vi "StateLED.vi"(0 "Master State In":T1(ring)) -> ()   [LabVIEW 2023]
doc: "This VI manages the apperance of the LEDs. The LED coloration and blink pattern report the robot mode and status. See project documentation for details."
uses:
  <vilib>/Rock Robotics/WPI/DriverStation/WPI_DriverStationRobotMode2.ctl
  GlobalMiscellaneous.vi
  GlobalDriverStationData.vi
  GlobalNoteHandling.vi
  GlobalElevator.vi
  GlobalShooter.vi
  GlobalDrivebase.vi
  GlobalAutonomous.vi
  GlobalPoseAndTargeting.vi
  <vilib>/vision/NI_Vision_Development_Module.lvlib
panel:
  in  "Shooter Ready Indication color":u32(colorbox)
  in  "Climb Background":u32(colorbox)=16717311
  in  "Speaker Background":u32(colorbox)=16717311
  in  "Amp Background":u32(colorbox)=16717311
  in  "Stow Background":u32(colorbox)=16717311
  in  "Human Control":u32(colorbox)=65280
  in  "Master Caution":u32(colorbox)=16736256
  in  "User Value Choice":u8(slide)=255 step=1 scale=0.0..255.0
  in  "User Saturation Choice":u8(slide)=255 step=1 scale=0.0..255.0
  in  "Pressure Insert":u32(colorbox)=91
  in  "Battery Insert":u32(colorbox)=65282
  in  "Pressure Background":u32(colorbox)=16711680
  in  "Battery Background":u32(colorbox)=16711680
  in  "Pressure LED Length":i32=6
  in  "Battery LED Length":i32=6
  in  "Battery Index":i32=4
  in  "Pressure Index":i32=4
  in  "Swerve 2 LED Index":i32
  in  "Swerve 3 LED Index":i32
  in  "Swerve 0 LED Index":i32=18
  in  "Swerve LED Length":i32=2
  in  "Swerve 1 LED Index":i32=18
  in  "Locate LED":bool
  in  "LED Index":i32
  out "User Blue":u8
  out "User Green":u8=255
  out "User Red":u8
  in  "Choose Hue":bool
  in  "User Hue Choice":u8(slide)=255 step=1 scale=0.0..255.0
  in  "Nominal":u32(colorbox)=65280
  in  "Master Alarm":u32(colorbox)=16711680
  in  "Robot Control":u32(colorbox)=16727040
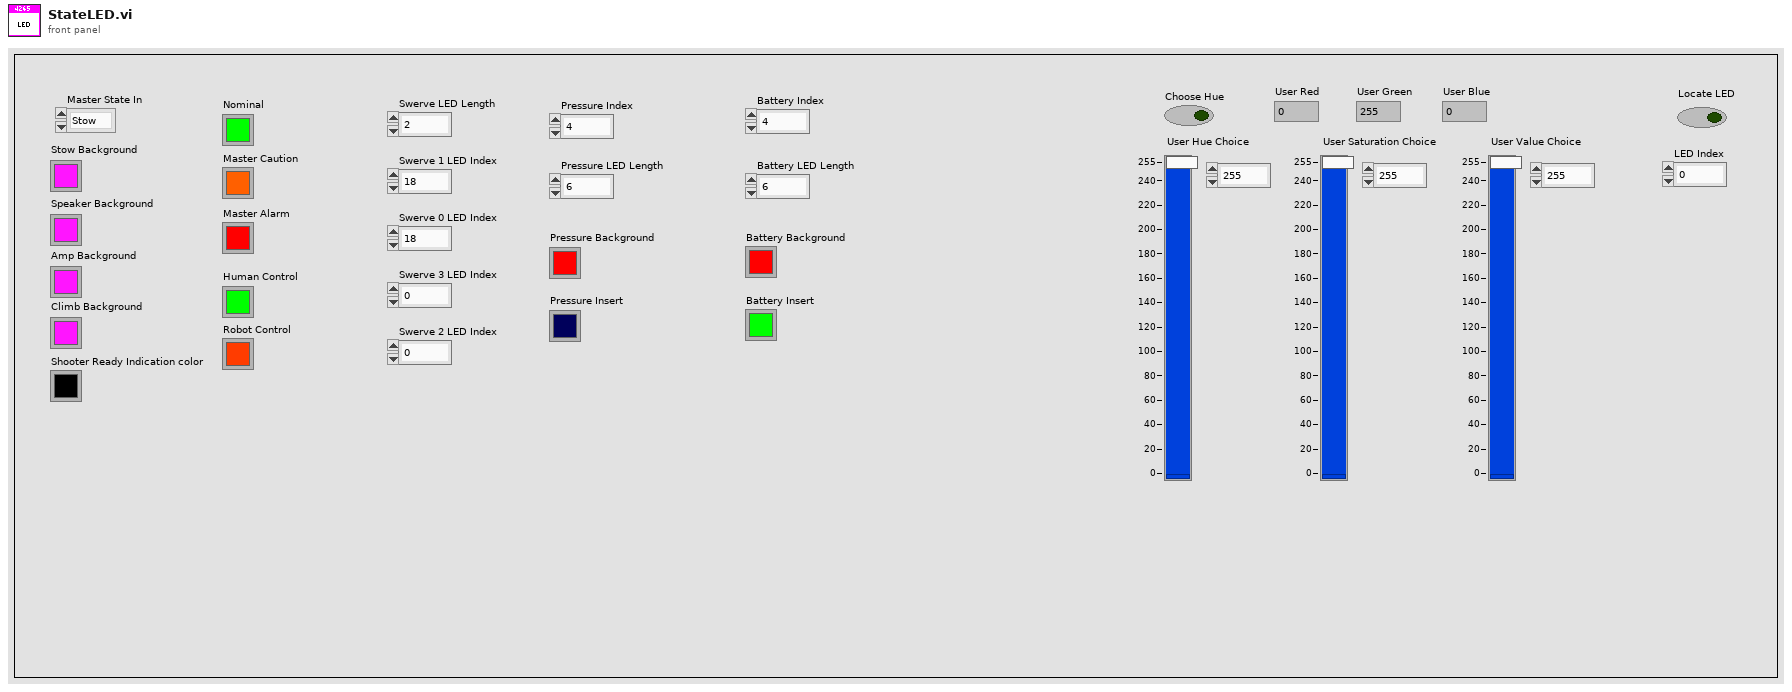
[diagram p1: front panel]
types:
  T1 = enum16{"Stow", "Speaker", "Amp", "Climbing", "Trap"}
  T2 = enum16{"Normal", "Party Mode", "Choose Hue", "Debug", "Locate LED", "Distance Rainbow"}
  T3 = typedef "WPI_DriverStationRobotMode2.ctl" = enum16{"Autonomous Disabled", "Autonomous Enabled", "Teleop Disabled", "Teleop Enabled", "Disconnected", "Finish", "Test Disabled", "Test Enabled", "Emergency Stopped"}
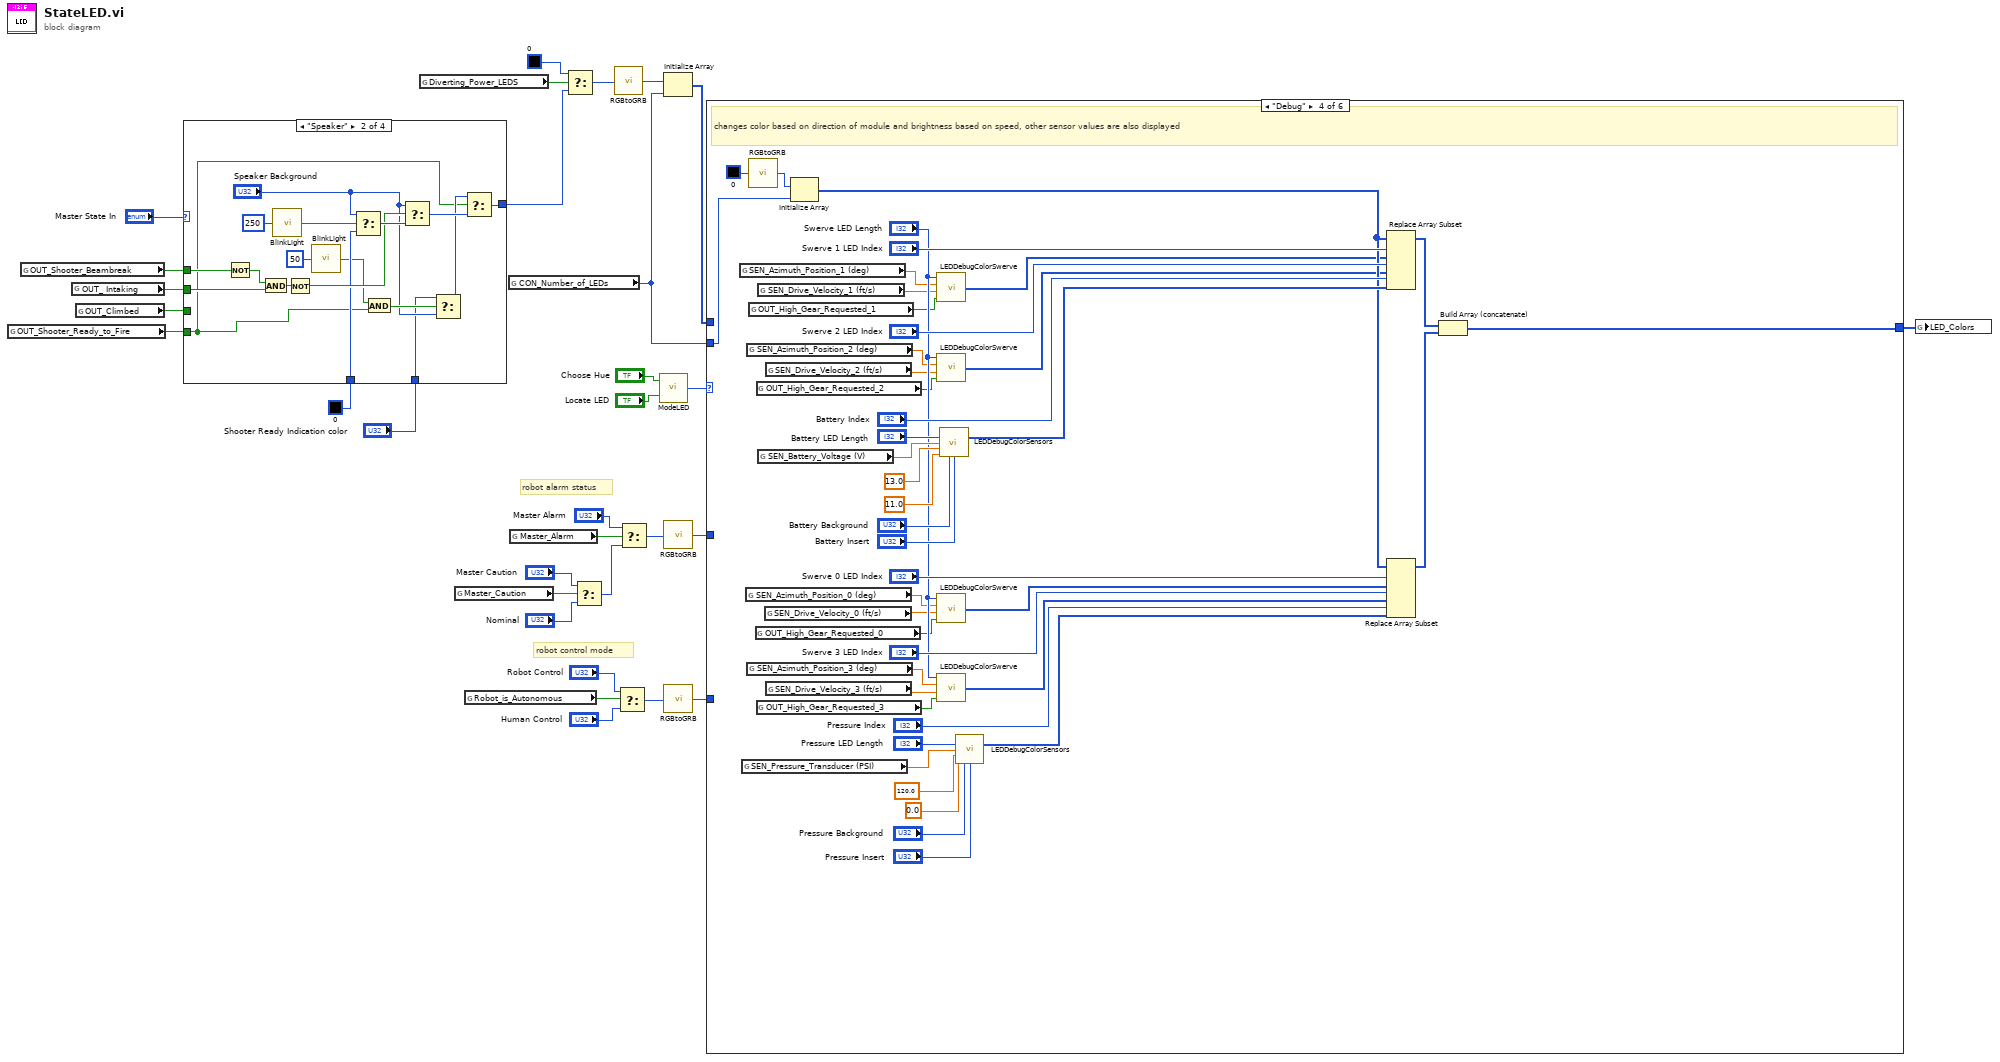
[diagram p0: block diagram]
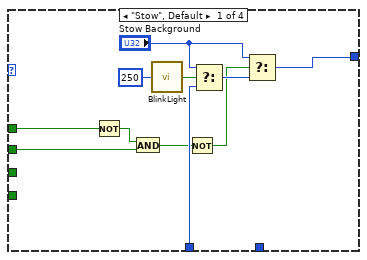
[diagram p2: hidden frame]
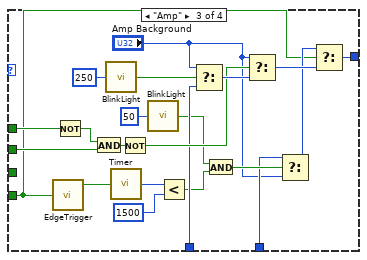
[diagram p3: hidden frame]
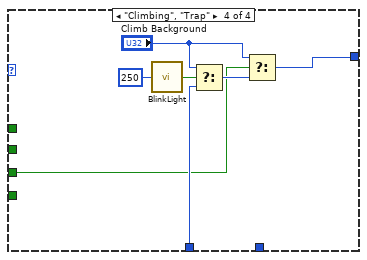
[diagram p4: hidden frame]
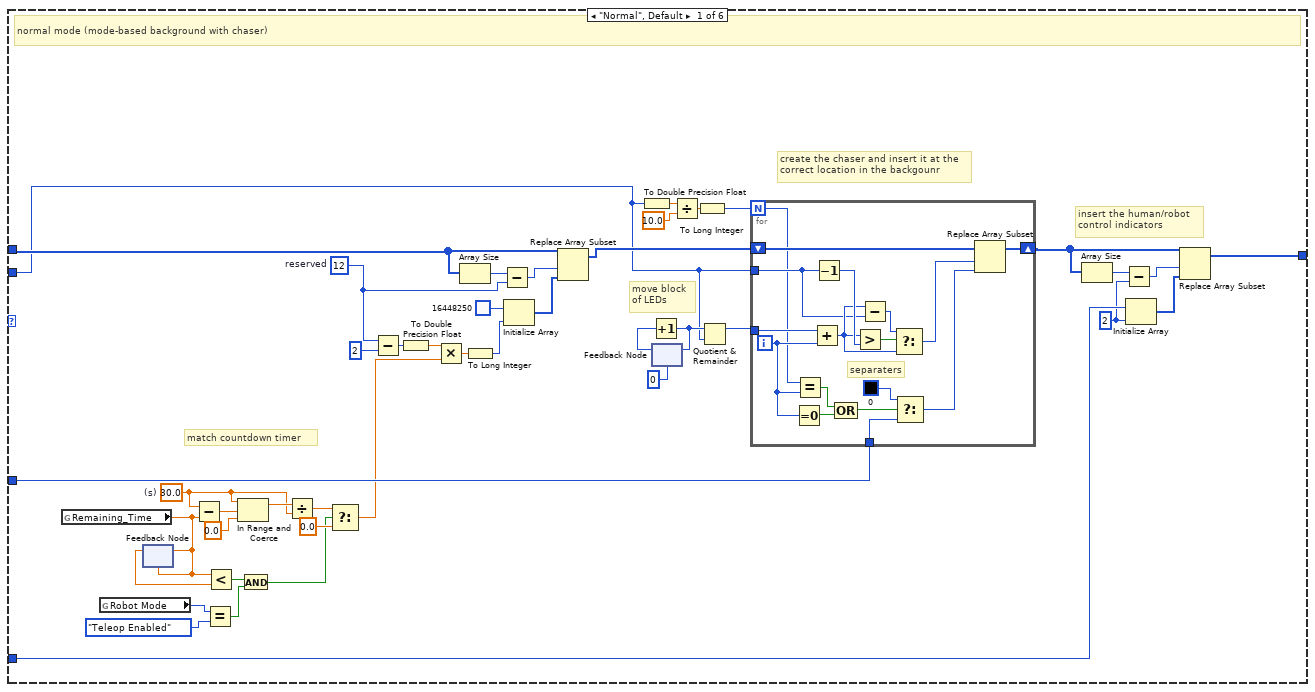
[diagram p5: hidden frame]
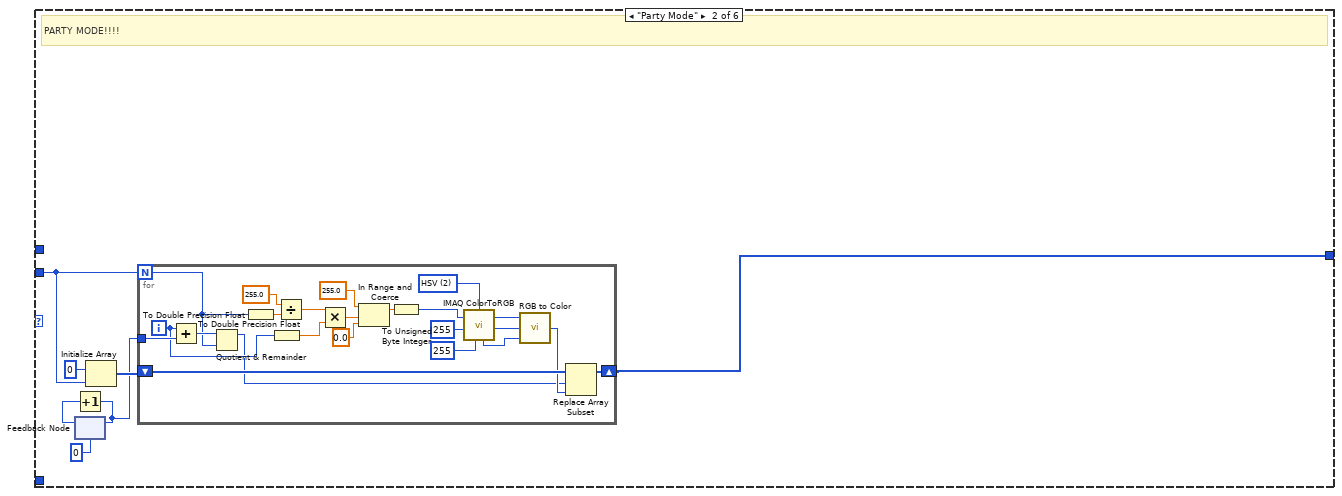
[diagram p6: hidden frame]
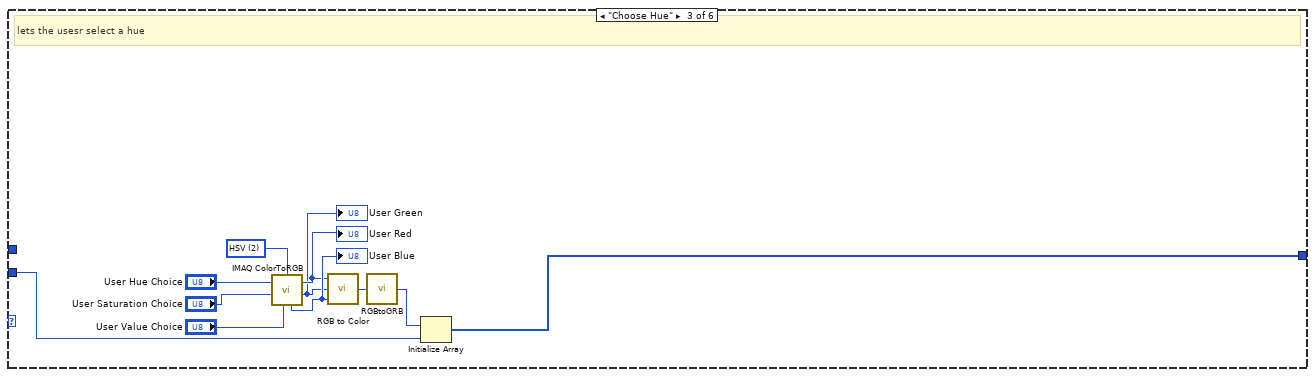
[diagram p7: hidden frame]
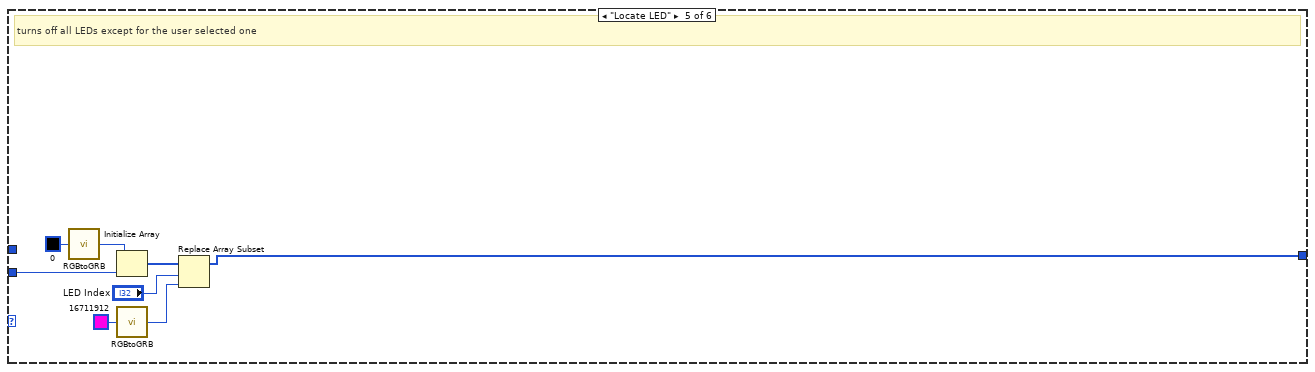
[diagram p8: hidden frame]
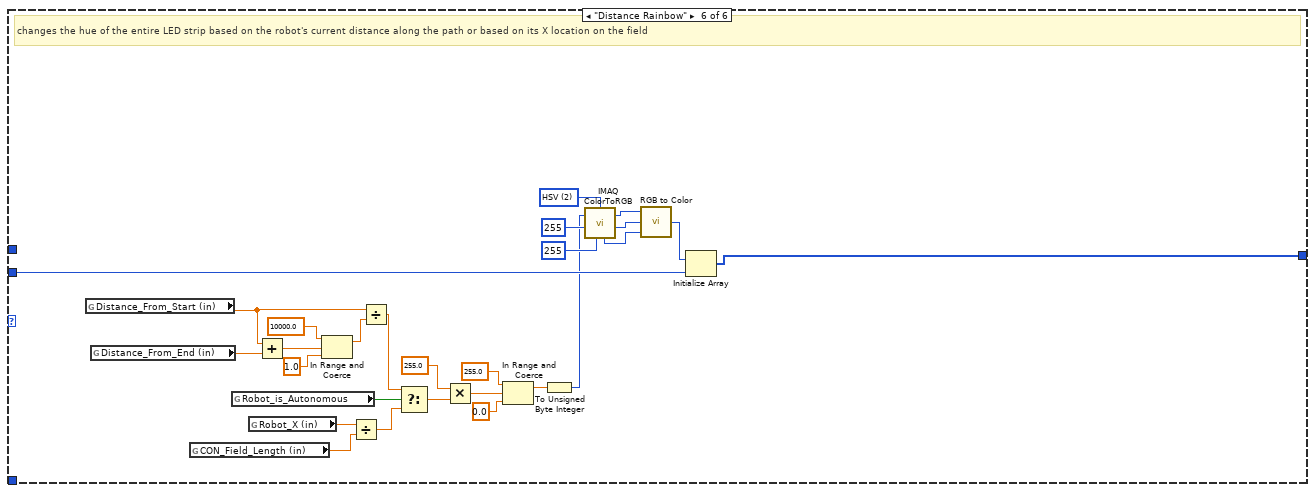
[diagram p9: hidden frame]
diagram:
  # "robot control mode"
  # "robot alarm status"
  n1 = global read "GlobalShooter.vi" "OUT_Shooter_Ready_to_Fire"() -> (w2:bool)
  n2 = global read "GlobalNoteHandling.vi" "OUT_Shooter_Beambreak"() -> (w5:bool)
  n3 = global read "GlobalNoteHandling.vi" "OUT_ Intaking"() -> (w4:bool)
  n4 = global read "GlobalElevator.vi" "OUT_Climbed"() -> (w3:bool)
  n5 = case shown="\"Speaker\"" "Master State In" {
    tunnel: [w37 w44 w62 w86] -> w7
    tunnel: u32 0 ("Diverting Power") -> [w40 w54 w76 w84]
    tunnel: w5 -> [w36 w52 w74 _]
    tunnel: w4 -> [w34 w53 w75 _]
    tunnel: w3 -> [_ _ _ w83]
    tunnel: w2 -> [_ w43 w63 _]
    tunnel: "Shooter Ready Indication color" -> [_ w47 w66 _]
    frame "Stow", Default {
      n6 = Not(x=w36) -> (.not. x?=w35:bool)
      n7 = And(x=w35, y=w34) -> (x .and. y?=w33:bool)
      n8 = call "BlinkLight.vi"("Blink Interval (ms)"=u32 250) -> ("Blinked Output"=w41:bool)
      n9 = Not(x=w33) -> (.not. x?=w32:bool)
      n10 = Select(t="Stow Background", s=w41, f=w40) -> (s? t:f=w38:u32)
      n11 = Select(t="Stow Background", s=w32, f=w38) -> (s? t:f=w37:u32)
    }
    frame "Speaker" {
      n12 = Not(x=w52) -> (.not. x?=w57:bool)
      n13 = And(x=w57, y=w53) -> (x .and. y?=w56:bool)
      n14 = call "BlinkLight.vi"("Blink Interval (ms)"=u32 250) -> ("Blinked Output"=w59:bool)
      n15 = Not(x=w56) -> (.not. x?=w55:bool)
      n16 = call "BlinkLight.vi"("Blink Interval (ms)"=u32 50) -> ("Blinked Output"=w50:bool)
      n17 = Select(t="Speaker Background", s=w59, f=w54) -> (s? t:f=w58:u32)
      n18 = And(x=w50, y=w43) -> (x .and. y?=w49:bool)
      n19 = Select(t="Speaker Background", s=w55, f=w58) -> (s? t:f=w46:u32)
      n20 = Select(t=w47, s=w49, f="Speaker Background") -> (s? t:f=w45:u32)
      n21 = Select(t=w45, s=w43, f=w46) -> (s? t:f=w44:u32)
    }
    frame "Amp" {
      n22 = call "EdgeTrigger.vi"("Input Signal"=w63) -> ("Rising Edge Trigger"=w72:bool)  [unwired: 2 out]
      n23 = Not(x=w74) -> (.not. x?=w79:bool)
      n24 = And(x=w79, y=w75) -> (x .and. y?=w78:bool)
      n25 = call "BlinkLight.vi"("Blink Interval (ms)"=u32 250) -> ("Blinked Output"=w81:bool)
      n26 = call "Timer.vi"("Reset Timer"=w72) -> ("Time (ms)"=w71:u32)
      n27 = Not(x=w78) -> (.not. x?=w77:bool)
      n28 = call "BlinkLight.vi"("Blink Interval (ms)"=u32 50) -> ("Blinked Output"=w69:bool)
      n29 = Less?(x=w71, y=u32 1500) -> (x < y?=w68:bool)
      n30 = Select(t="Amp Background", s=w81, f=w76) -> (s? t:f=w80:u32)
      n31 = And(x=w69, y=w68) -> (x .and. y?=w67:bool)
      n32 = Select(t="Amp Background", s=w77, f=w80) -> (s? t:f=w65:u32)
      n33 = Select(t=w66, s=w67, f="Amp Background") -> (s? t:f=w64:u32)
      n34 = Select(t=w64, s=w63, f=w65) -> (s? t:f=w62:u32)
    }
    frame "Climbing", "Trap" {
      n35 = call "BlinkLight.vi"("Blink Interval (ms)"=u32 250) -> ("Blinked Output"=w88:bool)
      n36 = Select(t="Climb Background", s=w88, f=w84) -> (s? t:f=w87:u32)
      n37 = Select(t="Climb Background", s=w83, f=w87) -> (s? t:f=w86:u32)
    }
  }
  n38 = global read "GlobalMiscellaneous.vi" "Diverting_Power_LEDS"() -> (w23:bool)
  n39 = global read "GlobalMiscellaneous.vi" "Master_Caution"() -> (w16:bool)
  n40 = global read "GlobalDriverStationData.vi" "Robot_is_Autonomous"() -> (w21:bool)
  n41 = global read "GlobalMiscellaneous.vi" "CON_Number_of_LEDs"() -> (w9:u16)
  n42 = global read "GlobalMiscellaneous.vi" "Master_Alarm"() -> (w22:bool)
  n43 = Select(t=u32 0 ("Diverting Power"), s=w23, f=w7) -> (s? t:f=w11:u32)
  n44 = Select(t="Master Caution", s=w16, f="Nominal") -> (s? t:f=w15:u32)
  n45 = call "RGBtoGRB.vi"("Color (RGB)"=w11) -> ("Color (GRB)"=w31:u32)
  n46 = Select(t="Robot Control", s=w21, f="Human Control") -> (s? t:f=w20:u32)
  n47 = Select(t="Master Alarm", s=w22, f=w15) -> (s? t:f=w18:u32)
  n48 = call "ModeLED.vi"("Locate LED"="Locate LED", "Choose Hue"="Choose Hue") -> ("LED Mode"=w26:T2)
  n49 = Initialize Array(w31, w9) -> (w28:u32[])
  n50 = call "RGBtoGRB.vi"("Color (RGB)"=w18) -> ("Color (GRB)"=w17:u32)
  n51 = call "RGBtoGRB.vi"("Color (RGB)"=w20) -> ("Color (GRB)"=w27:u32)
  n52 = case shown="\"Debug\"" w26 {
    tunnel: w28 -> [w110 _ _ _ _ _]
    tunnel: [w90 w150 w180 w217 w235 w243] -> w10
    tunnel: w27 -> [w132 _ _ _ _ _]
    tunnel: w9 -> [w98 w152 w187 w233 w236 w262]
    tunnel: w17 -> [w101 _ _ _ _ _]
    frame "Normal", Default {
      w119 = 30.0  # (s)
      w112 = 12  # reserved
      w130 = 2 ("dimension size")
      # "create the chaser and insert it at the \ncorrect location in the backgounr"
      # "move block\nof LEDs"
      # "match countdown timer"
      # "insert the human/robot\ncontrol indicators"
      # "normal mode (mode-based background with chaser)"
      n53 = global read "GlobalDriverStationData.vi" "Remaining_Time"() -> (w96:dbl)
      n54 = global read "GlobalDriverStationData.vi" "Robot Mode"() -> (w115:T3)
      n55 = feedback-in #1(w96) -> ()
      n56 = feedback #1(w96) -> (w97:dbl)
      n57 = Subtract(x=w119, y=w96) -> (x-y=w120:dbl)
      n58 = Equal?(x=w115, y=WPI_DriverStationRobotMode2."Teleop Enabled") -> (x = y?=w93:bool)
      n59 = Less?(x=w96, y=w97) -> (x < y?=w95:bool)
      n60 = In Range and Coerce(upper limit=w119, x=w120, lower limit=0.0) -> (coerced(x)=w121:dbl)  [unwired: 1 out]
      n61 = And(x=w95, y=w93) -> (x .and. y?=w94:bool)
      n62 = Divide(x=w121, y=w119) -> (x/y=w118:dbl)
      n63 = Select(t=w118, s=w94, f=0.0) -> (s? t:f=w91:dbl)
      n64 = Subtract(x=w112, y=2) -> (x-y=w113:i32)
      n65 = To Double Precision Float(number=w113) -> (double precision float=w124:dbl)
      n66 = Multiply(x=w124, y=w91) -> (x*y=w123:dbl)
      n67 = Array Size(array=w110) -> (size(s)=w127:i32)
      n68 = To Long Integer(number=w123) -> (32bit integer=w122:i32)
      n69 = Subtract(x=w127, y=w112) -> (x-y=w126:i32)
      n70 = Initialize Array(u32 16448250 ("Color"), w122) -> (w125:u32[])
      n71 = Replace Array Subset(array=w110, new element=w125, index=w126) -> (w99:u32[])
      n72 = To Double Precision Float(number=w98) -> (double precision float=w109:dbl)
      n73 = feedback #2(0) -> (w104:i32)
      n74 = Increment(x=w104) -> (x+1=w103:i32)
      n75 = feedback-in #2(w103) -> ()
      n76 = Divide(x=w109, y=10.0) -> (x/y=w108:dbl)
      n77 = To Long Integer(number=w108) -> (32bit integer=w100:i32)
      n78 = Quotient & Remainder(x=w103, y=w98) -> (x-y*floor(x/y)=w106:i32)  [unwired: 1 out]
      n79 = for {
        N: w100 -> [w133]
        tunnel: w106 -> [w149]
        tunnel: w98 -> [w142]
        shift-right: [w144] -> w102
        shift-left: w99 -> [w145]
        tunnel: w101 -> [w139]
        i -> [w134]
        # "separaters"
        n80 = Equal To 0?(x=w134) -> (x = 0?=w137:bool)
        n81 = Equal?(x=w133, y=w134) -> (x = y?=w135:bool)
        n82 = Add(x=w149, y=w134) -> (x+y=w143:i32)
        n83 = Decrement(x=w142) -> (x-1=w148:u16)
        n84 = Compound Arithmetic op=OR(w135, w137) -> (w136:bool)
        n85 = Greater?(x=w143, y=w148) -> (0:w147:bool)
        n86 = Subtract(x=w143, y=w142) -> (x-y=w141:i32)
        n87 = Select(t=w141, s=w147, f=w143) -> (s? t:f=w146:i32)
        n88 = Select(t=u32 0 ("Color (RGB)"), s=w136, f=w139) -> (s? t:f=w138:u32)
        n89 = Replace Array Subset(array=w145, new element=w138, index=w146) -> (w144:u32[])
      }
      n90 = Array Size(array=w102) -> (size(s)=w131:i32)
      n91 = Subtract(x=w131, y=w130) -> (x-y=w129:i32)
      n92 = Initialize Array(w132, w130) -> (w128:u32[])
      n93 = Replace Array Subset(array=w102, new element=w128, index=w129) -> (w90:u32[])
    }
    frame "Party Mode" {
      # "PARTY MODE!!!!"
      n94 = feedback #3(0) -> (w154:i32)
      n95 = Increment(x=w154) -> (x+1=w151:i32)
      n96 = feedback-in #3(w151) -> ()
      n97 = Initialize Array(u32 0 ("element"), w152) -> (w155:u32[])
      n98 = for {
        N: w152 -> [w159]
        shift-right: [w167] -> w150
        shift-left: w155 -> [w168]
        tunnel: w151 -> [w161]
        i -> [w158]
        w177 = u16 2 items=["RGB", "HSL", "HSV", "HSI"] ("Color Mode")
        n99 = Add(x=w158, y=w161) -> (x+y=w160:i32)
        n100 = Quotient & Remainder(x=w160, y=w159) -> (x-y*floor(x/y)=w157:i32)  [unwired: 1 out]
        n101 = To Double Precision Float(number=w159) -> (double precision float=w176:dbl)
        n102 = To Double Precision Float(number=w158) -> (double precision float=w173:dbl)
        n103 = Divide(x=255.0, y=w176) -> (x/y=w174:dbl)
        n104 = Multiply(x=w174, y=w173) -> (x*y=w172:dbl)
        n105 = In Range and Coerce(upper limit=255.0, x=w172, lower limit=0.0) -> (coerced(x)=w169:dbl)  [unwired: 1 out]
        n106 = To Unsigned Byte Integer(number=w169) -> (unsigned 8bit integer=w162:u8)
        n107 = call "IMAQ ColorToRGB"("Green or Sat value"=u8 255, "Blue or Luma or Val or Inten value"=u8 255, "Red or Hue value"=w162, "Color Mode"=w177) -> ("Blue value"=w163:u8, "Green value"=w164:u8, "Red value"=w165:u8)  [unwired: 1 in, 1 out]
        n108 = call <vilib>:"RGB to Color.vi"("B"=w163, "G"=w164, "R"=w165) -> ("Color"=w166:u32)
        n109 = Replace Array Subset(array=w168, new element=w166, index=w157) -> (w167:u32[])
      }
    }
    frame "Choose Hue" {
      w188 = u16 2 items=["RGB", "HSL", "HSV", "HSI"] ("Color Mode")
      # "lets the usesr select a hue"
      n110 = call "IMAQ ColorToRGB"("Green or Sat value"="User Saturation Choice", "Blue or Luma or Val or Inten value"="User Value Choice", "Red or Hue value"="User Hue Choice", "Color Mode"=w188) -> ("Blue value"=w189:u8, "Green value"=w183:u8, "Red value"=w184:u8)  [unwired: 1 in, 1 out]
      "User Red" <- w184
      "User Green" <- w183
      "User Blue" <- w189
      n111 = call <vilib>:"RGB to Color.vi"("B"=w189, "G"=w183, "R"=w184) -> ("Color"=w182:u32)
      n112 = call "RGBtoGRB.vi"("Color (RGB)"=w182) -> ("Color (GRB)"=w181:u32)
      n113 = Initialize Array(w181, w187) -> (w180:u32[])
    }
    frame "Debug" {
      # "changes color based on direction of module and brightness based on speed, other sensor values are also displayed"
      n114 = global read "GlobalDrivebase.vi" "SEN_Azimuth_Position_1 (deg)"() -> (w202:dbl)
      n115 = global read "GlobalMiscellaneous.vi" "SEN_Pressure_Transducer (PSI)"() -> (w222:dbl)
      n116 = global read "GlobalDrivebase.vi" "SEN_Azimuth_Position_0 (deg)"() -> (w197:dbl)
      n117 = global read "GlobalDrivebase.vi" "SEN_Azimuth_Position_2 (deg)"() -> (w199:dbl)
      n118 = global read "GlobalDrivebase.vi" "SEN_Azimuth_Position_3 (deg)"() -> (w194:dbl)
      n119 = call "RGBtoGRB.vi"("Color (RGB)"=u32 0) -> ("Color (GRB)"=w219:u32)
      n120 = global read "GlobalDrivebase.vi" "OUT_High_Gear_Requested_1"() -> (w191:bool)
      n121 = global read "GlobalDrivebase.vi" "OUT_High_Gear_Requested_0"() -> (w195:bool)
      n122 = global read "GlobalDrivebase.vi" "OUT_High_Gear_Requested_2"() -> (w198:bool)
      n123 = global read "GlobalDrivebase.vi" "OUT_High_Gear_Requested_3"() -> (w192:bool)
      n124 = global read "GlobalDrivebase.vi" "SEN_Drive_Velocity_1 (ft/s)"() -> (w201:dbl)
      n125 = global read "GlobalMiscellaneous.vi" "SEN_Battery_Voltage (V)"() -> (w221:dbl)
      n126 = global read "GlobalDrivebase.vi" "SEN_Drive_Velocity_0 (ft/s)"() -> (w196:dbl)
      n127 = global read "GlobalDrivebase.vi" "SEN_Drive_Velocity_2 (ft/s)"() -> (w200:dbl)
      n128 = global read "GlobalDrivebase.vi" "SEN_Drive_Velocity_3 (ft/s)"() -> (w193:dbl)
      n129 = Initialize Array(w219, w233) -> (w213:u32[])
      n130 = call "LEDDebugColorSwerve.vi"("Shifter State"=w191, "Drive Velocity (ft/s)"=w201, "Azimuth Angle (deg [-180,180])"=w202, "Swerve LED Length"="Swerve LED Length") -> ("Color Array"=w207:u32[])
      n131 = call "LEDDebugColorSwerve.vi"("Shifter State"=w198, "Drive Velocity (ft/s)"=w200, "Azimuth Angle (deg [-180,180])"=w199, "Swerve LED Length"="Swerve LED Length") -> ("Color Array"=w206:u32[])
      n132 = call "LEDDebugColorSwerve.vi"("Shifter State"=w195, "Drive Velocity (ft/s)"=w196, "Azimuth Angle (deg [-180,180])"=w197, "Swerve LED Length"="Swerve LED Length") -> ("Color Array"=w205:u32[])
      n133 = call "LEDDebugColorSwerve.vi"("Shifter State"=w192, "Drive Velocity (ft/s)"=w193, "Azimuth Angle (deg [-180,180])"=w194, "Swerve LED Length"="Swerve LED Length") -> ("Color Array"=w204:u32[])
      n134 = call "LEDDebugColorSensors.vi"("LED Length"="Battery LED Length", "Value"=w221, "Max"=13.0, "Min"=11.0, "Background Color"="Battery Background", "Color to Insert"="Battery Insert") -> ("Output Color Array"=w214:u32[])  [unwired: 9 in]
      n135 = call "LEDDebugColorSensors.vi"("LED Length"="Pressure LED Length", "Value"=w222, "Max"=120.0, "Min"=0.0, "Background Color"="Pressure Background", "Color to Insert"="Pressure Insert") -> ("Output Color Array"=w208:u32[])  [unwired: 9 in]
      n136 = Replace Array Subset(array=w213, new element #1=w207, index #1="Swerve 1 LED Index", new element #2=w206, index #2="Swerve 2 LED Index", new element #3=w214, index #3="Battery Index") -> (w218:u32[])
      n137 = Replace Array Subset(array=w213, new element #1=w205, index #1="Swerve 0 LED Index", new element #2=w204, index #2="Swerve 3 LED Index", new element #3=w208, index #3="Pressure Index") -> (w212:u32[])
      n138 = Build Array (concatenate)(w218, w212) -> (w217:u32[])
    }
    frame "Locate LED" {
      # "turns off all LEDs except for the user selected one"
      n139 = call "RGBtoGRB.vi"("Color (RGB)"=u32 0) -> ("Color (GRB)"=w241:u32)
      n140 = Initialize Array(w241, w236) -> (w240:u32[])
      n141 = call "RGBtoGRB.vi"("Color (RGB)"=u32 16711912) -> ("Color (GRB)"=w238:u32)
      n142 = Replace Array Subset(array=w240, new element=w238, index="LED Index") -> (w235:u32[])
    }
    frame "Distance Rainbow" {
      w266 = u16 2 items=["RGB", "HSL", "HSV", "HSI"] ("Color Mode")
      # "changes the hue of the entire LED strip based on the robot's current distance along the path or based on its X location on the field"
      n143 = global read "GlobalAutonomous.vi" "Distance_From_Start (in)"() -> (w256:dbl)
      n144 = global read "GlobalAutonomous.vi" "Distance_From_End (in)"() -> (w261:dbl)
      n145 = global read "GlobalPoseAndTargeting.vi" "CON_Field_Length (in)"() -> (w244:dbl)
      n146 = global read "GlobalDriverStationData.vi" "Robot_is_Autonomous"() -> (w245:bool)
      n147 = global read "GlobalPoseAndTargeting.vi" "Robot_X (in)"() -> (w251:dbl)
      n148 = Add(x=w256, y=w261) -> (x+y=w260:dbl)
      n149 = In Range and Coerce(upper limit=10000.0 ("x"), x=w260, lower limit=1.0) -> (coerced(x)=w257:dbl)  [unwired: 1 out]
      n150 = Divide(x=w251, y=w244) -> (x/y=w246:dbl)
      n151 = Divide(x=w256, y=w257) -> (x/y=w255:dbl)
      n152 = Select(t=w255, s=w245, f=w246) -> (s? t:f=w254:dbl)
      n153 = Multiply(x=255.0, y=w254) -> (x*y=w248:dbl)
      n154 = In Range and Coerce(upper limit=255.0 ("x"), x=w248, lower limit=0.0) -> (coerced(x)=w247:dbl)  [unwired: 1 out]
      n155 = To Unsigned Byte Integer(number=w247) -> (unsigned 8bit integer=w252:u8)
      n156 = call "IMAQ ColorToRGB"("Green or Sat value"=u8 255 ("User Saturation Choice 2"), "Blue or Luma or Val or Inten value"=u8 255 ("User Value Choice 2"), "Red or Hue value"=w252, "Color Mode"=w266) -> ("Blue value"=w269:u8, "Green value"=w268:u8, "Red value"=w267:u8)  [unwired: 1 in, 1 out]
      n157 = call <vilib>:"RGB to Color.vi"("B"=w269, "G"=w268, "R"=w267) -> ("Color"=w265:u32)
      n158 = Initialize Array(w265, w262) -> (w243:u32[])
    }
  }
  n159 = global write "GlobalMiscellaneous.vi" "LED_Colors"(w10) -> ()
